vi "Help.vi"() -> ()   [LabVIEW 2013]
panel:
  in  "OK Button":bool
  # "Proceso de calibración:\n\nPuesta a cero. - Retirar el peso de calibración de la balanza.\nUna vez que la lectura de la casilla \"Lectura A/D\" sea estable, pulsar\nel botón \"Zero\". \nLa lectura de la balanza será ahora de 0.000 mg\n\nCalibración:- Colocar el peso de calibración en la balanza e introducir\nel peso correspondiente en la casilla \"Peso de calibración (mg)\".\nUna vez que la lectura de la casilla \"Lectura A/D\" sea estable, pulsar\nel botón \"Calibrate\". \nLa lectura de la balanza corresponderá al peso de calibración\n\nFinalizar calibración: - Quitar el peso de calibración de la balanza.\nLa lectura de la balanza debe retornar a 0.000 mg"
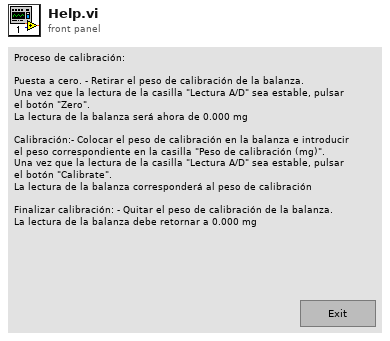
[diagram p1: front panel]
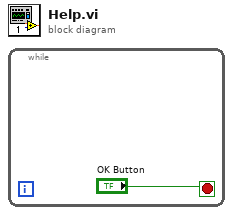
[diagram p0: block diagram]
diagram:
  n1 = while {
    stop <- "OK Button" stop-if-true
  }
